vi "Insert Single Event.vi"(4 "Insert?":bool, 5 "Event to insert":string, 7 "Event queue in":string[](array[string])) -> (3 "Event queue out":string[](array[string]))   [LabVIEW 2013]
doc: "Inserts an event or list of events into the event queue. Inserting is conditional based on the 'Insert' control."
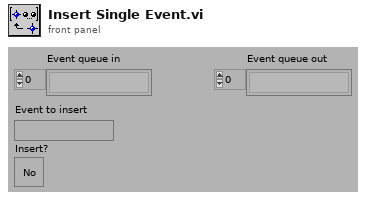
[diagram p1: front panel]
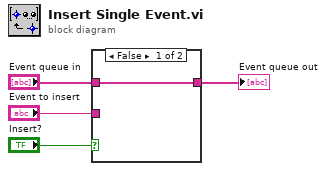
[diagram p0: block diagram]
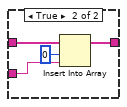
[diagram p2: hidden frame]
diagram:
  n1 = case shown="False" "Insert?" {
    tunnel: "Event to insert" -> [_ w8]
    tunnel: [w5 w7] -> w3
    tunnel: "Event queue in" -> [w5 w9]
    frame False {
    }
    frame True {
      n2 = Insert Into Array(array=w9, index=0 ("Index"), new element=w8) -> (w7:string[])
    }
  }
  "Event queue out" <- w3
